vi "DisplayHWTimedImages.vi"(0 "object in":refnum<class "Hamamatsu.lvclass">, 2 "HWSyncedImages":T1[](array[typedef]), 5 "error in (no error)":errorcluster) -> (14 "object out":refnum<class "Hamamatsu.lvclass">, 19 "error out":errorcluster)   [LabVIEW 2021, in "Hamamatsu.lvclass"]
uses:
  Hamamatsu.lvclass
  Hamamatsu.lvclass/Hamamatsu.ctl
  <vilib>/vision/Image Controls.llb/IMAQ Image.ctl
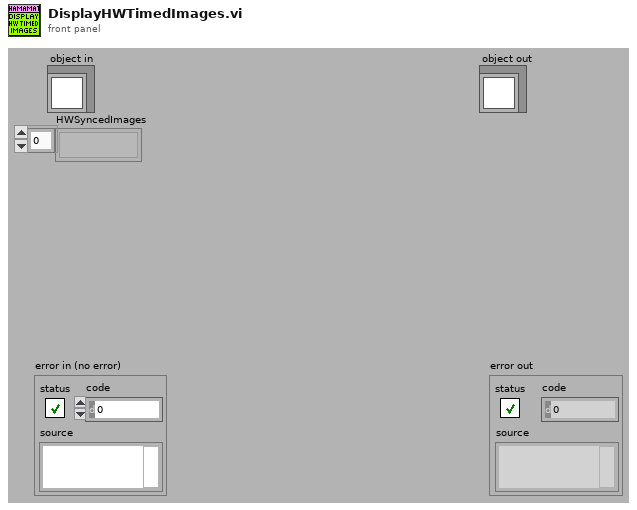
[diagram p1: front panel]
types:
  T1 = typedef "IMAQ Image.ctl" = refnum<image>
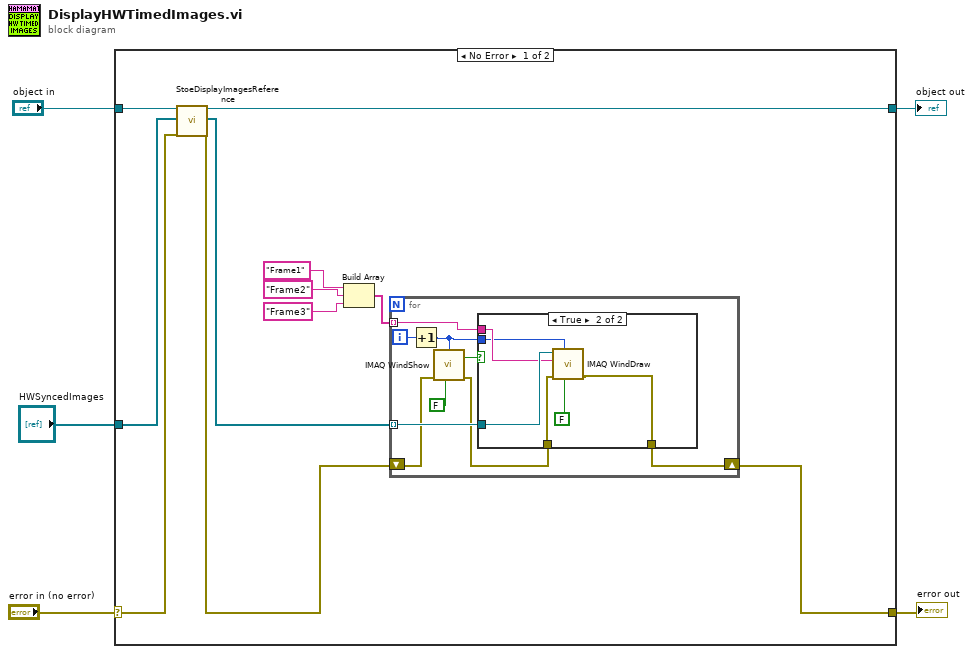
[diagram p0: block diagram]
diagram:
  n1 = case shown="No Error" "error in (no error)" {
    selector: "error in (no error)" -> [w7 w34]
    tunnel: [w12 w34] -> w4
    tunnel: [w11 w33] -> w2
    tunnel: "object in" -> [w10 w33]
    tunnel: "HWSyncedImages" -> [w8 _]
    frame No Error {
      n2 = call-dynamic "StoeDisplayImagesReference.vi"("object in"=w10, "Image Src"=w8, "error in (no error)"=w7) -> ("object out"=w11:refnum<class "Hamamatsu.lvclass">, "Images for Display Purpose"=w9:T1[], "error out"=w6:errorcluster)  [unwired: 14 in]
      n3 = Build Array("Frame1" ("Title"), "Frame2" ("Title"), "Frame3" ("Title")) -> (w14:string[])
      n4 = for {
        tunnel: w9 -> [w24] mode=indexing
        shift-right: [w17] -> w12
        shift-left: w6 -> [w23]
        tunnel: w14 -> [w19] mode=indexing
        i -> [w21]
        n5 = Increment(x=w21) -> (x+1=w20:i32)
        n6 = call "IMAQ WindShow"("error in (no error)"=w23, "Get/Set Status? (Set)"=FALSE, "Window Number (0...15)"=w20) -> ("error out"=w22:errorcluster, "Visible?"=w18:bool)  [unwired: 3 in, 1 out]
        n7 = case shown="True" w18 {
          tunnel: w24 -> [_ w31]
          tunnel: w22 -> [w26 w30]
          tunnel: w20 -> [_ w28]
          tunnel: w19 -> [_ w29]
          tunnel: [w26 w27] -> w17
          frame False {
          }
          frame True {
            n8 = call "IMAQ WindDraw"("Resize to Image Size? (Y)"=FALSE, "Window Number (0...15)"=w28, "error in (no error)"=w30, "Title"=w29, "Image"=w31) -> ("error out"=w27:errorcluster)  [unwired: 5 in, 1 out]
          }
        }
      }
    }
    frame Error {
    }
  }
  "error out" <- w4
  "object out" <- w2
